vi "ProgramStatus.vi"(0 "Universal Robot.lvclass in":refnum<class "Universal Robot.lvclass">, 5 "error in (no error)":errorcluster) -> (14 "Universal Robot.lvclass out":refnum<class "Universal Robot.lvclass">, 15 "Program Status":T1, 19 "error out":errorcluster)   [LabVIEW 2016, in "Universal Robot.lvclass"]
uses:
  Universal Robot.lvclass
  ProgramStatus.ctl
  ProgramState.ctl
  Universal Robot.lvclass/Universal Robot.ctl
  DashboardServer/Dashboard Server.lvclass
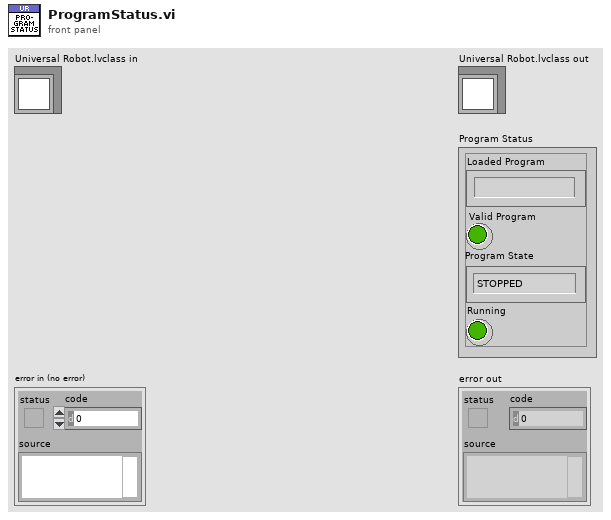
[diagram p1: front panel]
types:
  T1 = typedef "Universal Robot.lvclass/ProgramStatus.ctl" = cluster{"Loaded Program":string, "Valid Program":bool, "Program State":T2, "Running":bool}
  T2 = typedef "Universal Robot.lvclass/ProgramState.ctl" = enum16{"STOPPED", "PLAYING", "PAUSE"}
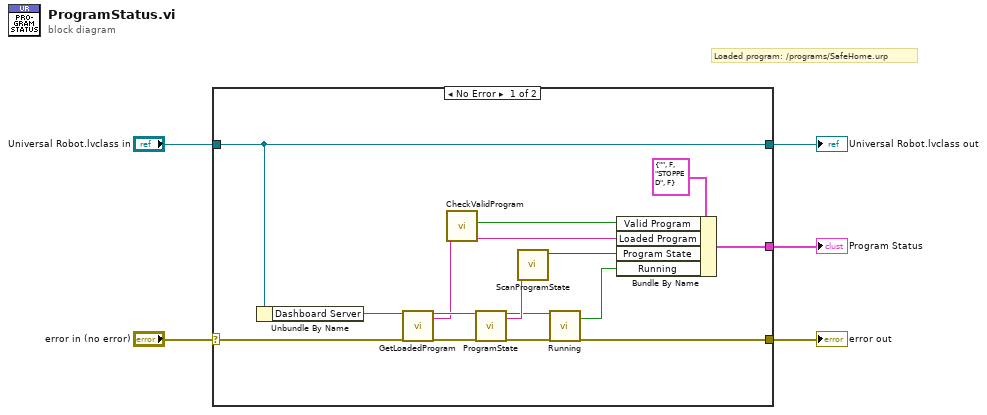
[diagram p0: block diagram]
diagram:
  # "Loaded program: /programs/SafeHome.urp"
  n1 = case shown="No Error" "error in (no error)" {
    selector: "error in (no error)" -> [w17 w23]
    tunnel: [w10 w23] -> w4
    tunnel: "Universal Robot.lvclass in" -> [w21 w22]
    tunnel: [w21 w22] -> w2
    tunnel: [w20 _] -> w1
    frame No Error {
      n2 = Unbundle By Name(w21) -> ("Dashboard Server"=w18:refnum<class "Dashboard Server.lvclass">)
      n3 = call-dynamic "GetLoadedProgram.vi"("DashboardServer in"=w18, "error in (no error)"=w17) -> ("DashboardServer out"=w16:refnum<class "Dashboard Server.lvclass">, "loadedProgram"=w8:string, "error out"=w15:errorcluster)  [unwired: 15 in]
      n4 = call "CheckValidProgram.vi"("loadedProgram in"=w8) -> ("loadedProgram out"=w7:string, "valid?"=w6:bool)  [unwired: 9 in]
      n5 = call-dynamic "ProgramState.vi"("DashboardServer in"=w16, "error in (no error)"=w15) -> ("DashboardServer out"=w12:refnum<class "Dashboard Server.lvclass">, "programState"=w14:string, "error out"=w11:errorcluster)  [unwired: 15 in]
      n6 = call "ScanProgramState.vi"("programState in"=w14) -> ("programState out"=w13:T2)  [unwired: 10 in]
      n7 = call-dynamic "Running.vi"("DashboardServer in"=w12, "error in (no error)"=w11) -> ("running"=w9:bool, "error out"=w10:errorcluster)  [unwired: 15 in, 1 out]
      n8 = Bundle By Name(cluster=T1 {"Loaded Program"="", "Valid Program"=FALSE, "Program State"=enum."STOPPED", "Running"=FALSE} ("Program Status"), "Valid Program"=w6, "Loaded Program"=w7, "Program State"=w13, "Running"=w9) -> (w20:T1)
    }
    frame Error {
    }
  }
  "error out" <- w4
  "Universal Robot.lvclass out" <- w2
  "Program Status" <- w1
